vi "Fields Remove Duplicates.vi"(8 "error in (no error)":errorcluster, 11 "Connection Refnum":T1) -> (0 "error out":errorcluster, 3 "Connection Refnum":T1)   [LabVIEW 2011]
uses:
  Summitek EXT/ODBC/SQL Controls/Connection Refnum.ctl
  Field Order By.ctl
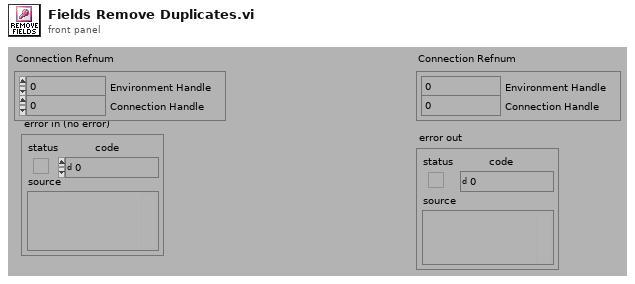
[diagram p1: front panel]
types:
  T1 = typedef "Connection Refnum.ctl" = cluster{"Environment Handle":i32, "Connection Handle":i32}
  T2 = cluster{"sxFieldId":string, "sxSequenceId":string}
  T3 = typedef "Field Order By.ctl" = enum32{"sxSequenceId", "sxFieldId", "sDisplayName", "sValue", "fSetAtTest", "fRequired", "nNextItem"}
  T4 = typedef "Field Record.ctl" = cluster{"ixField":i32, "iSequenceOrder":i32, "sxFieldId":string, "sxSequenceId":string, "sDisplayName":string, "sValue":string, "sUnits":string, "nDataType":T5, "nNextItem":T6, "fSystem":bool, "fSystemValue":bool, "fRequired":bool, "fSetAtTest":bool, "fTestField":bool, "fDeleted":bool, "fIndexed":bool, "fFreeList":bool}
  T5 = typedef "Field DataTypes.ctl" = enum32{"text", "numeric", "list", "timestamp", "boolean"}
  T6 = typedef "Field NextItem.ctl" = enum32{"Reset", "Retain", "Auto-Increment"}
  T7 = cluster{"sxFieldId":string, "sxSequenceId":string}[]
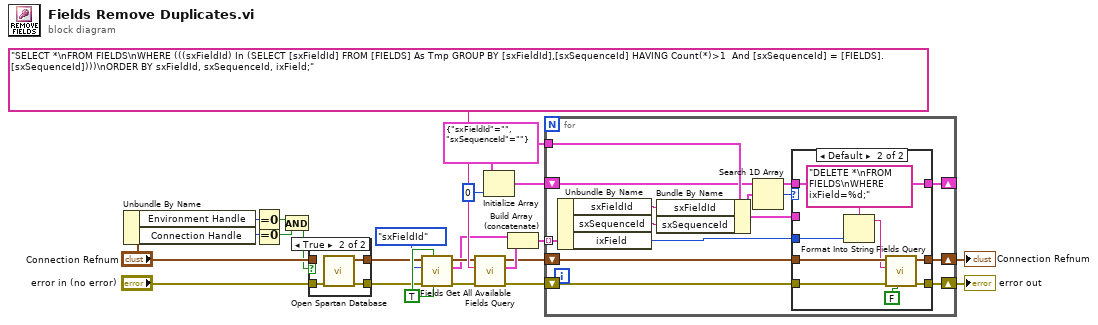
[diagram p0: block diagram]
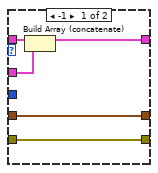
[diagram p3: hidden frame]
diagram:
  w12 = T2 {"sxFieldId"="", "sxSequenceId"=""}
  w21 = TRUE ("Combine All? (f)")
  n1 = Unbundle By Name("Connection Refnum") -> ("Environment Handle"=w4:i32, "Connection Handle"=w5:i32)
  n2 = Equal To 0?(x=w4) -> (x = 0?=w3:bool)
  n3 = Equal To 0?(x=w5) -> (x = 0?=w2:bool)
  n4 = And(x=w3, y=w2) -> (x .and. y?=w1:bool)
  n5 = case shown="True" w1 {
    tunnel: "error in (no error)" -> [w25 w29]
    tunnel: [w25 w28] -> w8
    tunnel: "Connection Refnum" -> [w26 _]
    tunnel: [w26 w27] -> w7
    frame False {
    }
    frame True {
      n6 = call "Open Spartan Database.vi"("error in (no error)"=w29) -> ("error out"=w28:errorcluster, "Connection Refnum"=w27:T1)  [unwired: 9 in]
    }
  }
  n7 = call "Fields Get All Available.vi"("Combine All? (f)"=w21, "Include Deleted? (F)"=w21, "error in (no error)"=w8, "Sort by (sxSequenceId)"=Field_Order_By."sxFieldId", "Connection Refnum"=w7) -> ("error out"=w22:errorcluster, "System or ALL Combined Fields"=w19:T4[], "Connection Refnum"=w23:T1)  [unwired: 1 in, 3 out]
  n8 = call "Fields Query.vi"("error in (no error)"=w22, "Query"="SELECT *\nFROM FIELDS\nWHERE (((sxFieldId) In (SELECT [sxFieldId] FROM [FIELDS] As Tmp GROUP BY [sxFieldId],[sxSequenceId] HAVING Count(*)>1  And [sxSequenceId] = [FIELDS].[sxSequenceId])))\nORDER BY sxFieldId, sxSequenceId, ixField;" ("User Query"), "Connection Refnum"=w23) -> ("error out"=w16:errorcluster, "Fields"=w18:T4[], "Connection Refnum"=w15:T1)  [unwired: 5 in, 1 out]
  n9 = Initialize Array(w12, 0 ("dimension size")) -> (w13:T7)
  n10 = Build Array (concatenate)(w19, w18) -> (w17:T4[])
  n11 = for {
    tunnel: w17 -> [w31] mode=indexing
    shift-right: [w33] -> w11
    shift-left: w16 -> [w34]
    shift-right: [w32] -> w10
    shift-left: w15 -> [w35]
    shift-right: [w36] -> _
    shift-left: w13 -> [w38]
    tunnel: w12 -> [w42]
    n12 = Unbundle By Name(w31) -> ("sxFieldId"=w41:string, "sxSequenceId"=w40:string, "ixField"=w30:i32)
    n13 = Bundle By Name(cluster=w42, "sxFieldId"=w41, "sxSequenceId"=w40) -> (w37:T2)
    n14 = Search 1D Array(1D array=w38, element=w37) -> (index of element=w39:i32)  [unwired: 1 in]
    n15 = case shown="Default" w39 {
      tunnel: w38 -> [w47 w56]
      tunnel: w37 -> [w46 _]
      tunnel: [w45 w56] -> w36
      tunnel: w35 -> [w43 w51]
      tunnel: w34 -> [w44 w54]
      tunnel: [w44 w53] -> w33
      tunnel: [w43 w52] -> w32
      tunnel: w30 -> [_ w49]
      frame -1 {
        n16 = Build Array (concatenate)(w47, w46) -> (w45:T7)
      }
      frame Default {
        n17 = Format Into String(format string="DELETE *\nFROM FIELDS\nWHERE ixField=%d;" ("User Query"), w49) -> (resulting string=w50:string)  [unwired: 2 in, 1 out]
        n18 = call "Fields Query.vi"("Return Data? (T)"=FALSE, "error in (no error)"=w54, "Query"=w50, "Connection Refnum"=w51) -> ("error out"=w53:errorcluster, "Connection Refnum"=w52:T1)  [unwired: 4 in, 2 out]
      }
    }
  }
  "error out" <- w11
  "Connection Refnum" <- w10
